vi "Apply Ethernet Configuration.vi"(7 "Restart (T)":bool=TRUE, 8 "error in (no error)":errorcluster, 10 "Ethernet Settings":T1={"IP Address"="192.168.1.100", "TCP (Command) Port"=12345, "TCP (Command) Read Interval (ms)"=10, "UDP (Reporting) Port"=54321, "UDP (Reporting) Write Interval (ms)"=5, "UDP Data Broadcast Enable"=FALSE}, 11 "Ethernet in":refnum<class "ENET_BS120x.lvclass">) -> (0 "error out":errorcluster, 3 "Ethernet out":refnum<class "ENET_BS120x.lvclass">)   [LabVIEW 2021, in "BS120x Driver.lvlib" / "ENET_BS120x.lvclass"]
doc: "Sends the configuration updates to the Battery Simulator 1200, and automatically triggers a restart.\nFor BS1201: the Restart input is no longer required. Restart is automatic on the BS1201 when configuration changes are made.\n(c) 2019 Bloomy Controls, Inc. All rights reserved."
uses:
  ENET_BS120x.lvclass
  TypeDefs/Ethernet Settings.ctl
  ENET_BS120x.lvclass/ENET_BS120x.ctl
  BS120x.lvclass
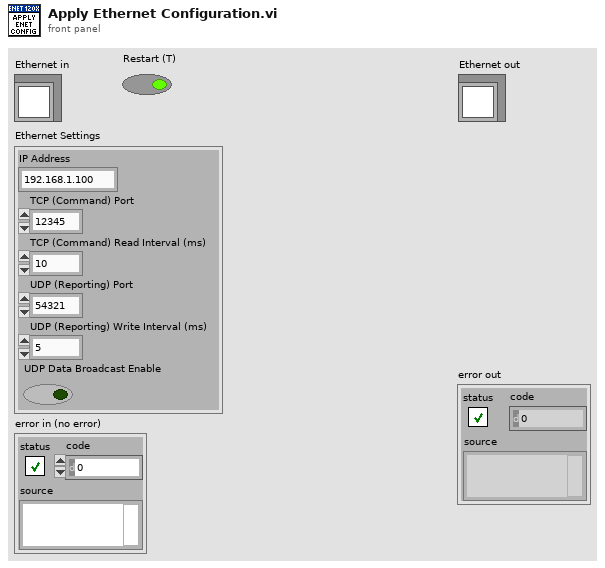
[diagram p1: front panel]
types:
  T1 = typedef "BS120x Driver.lvlib/BS120x.lvclass/Ethernet Settings.ctl" = cluster{"IP Address":string, "TCP (Command) Port":u16, "TCP (Command) Read Interval (ms)":u32, "UDP (Reporting) Port":u16, "UDP (Reporting) Write Interval (ms)":u32, "UDP Data Broadcast Enable":bool}
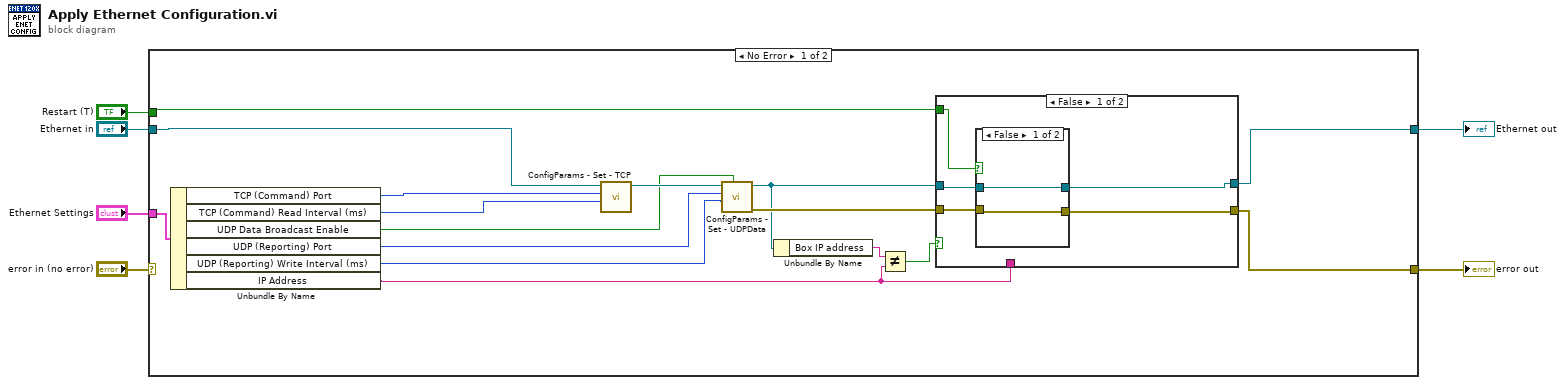
[diagram p0: block diagram]
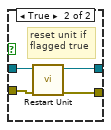
[diagram p2: hidden frame]
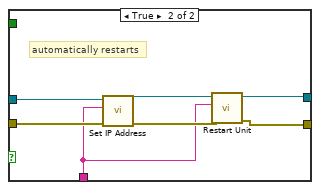
[diagram p3: hidden frame]
diagram:
  n1 = case shown="No Error" "error in (no error)" {
    selector: "error in (no error)" -> [_ w42]
    tunnel: [w13 w42] -> w5
    tunnel: [w12 w41] -> w3
    tunnel: "Ethernet in" -> [w21 w41]
    tunnel: "Ethernet Settings" -> [w22 _]
    tunnel: "Restart (T)" -> [w7 _]
    frame No Error {
      n2 = Unbundle By Name(w22) -> ("TCP (Command) Port"=w20:u16, "TCP (Command) Read Interval (ms)"=w19:u32, "UDP Data Broadcast Enable"=w16:bool, "UDP (Reporting) Port"=w17:u16, "UDP (Reporting) Write Interval (ms)"=w15:u32, "IP Address"=w9:string)
      n3 = call-dynamic "ConfigParams - Set - TCP.vi"("TCPLoopTime_mS"=w19, "TCPCommandPort"=w20, "Ethernet in"=w21) -> ("Ethernet out"=w18:refnum<class "ENET_BS120x.lvclass">)  [unwired: 7 in, 1 out]
      n4 = call-dynamic "ConfigParams - Set - UDPData.vi"("UDP Data Enable"=w16, "UDPDataPeriod_mS"=w15, "UDP Data Port"=w17, "Ethernet in"=w18) -> ("error out"=w14:errorcluster, "Ethernet out"=w11:refnum<class "ENET_BS120x.lvclass">)  [unwired: 6 in]
      n5 = Unbundle By Name(w11) -> ("Box IP address"=w10:string)
      n6 = Not Equal?(x=w10, y=w9) -> (x != y?=w8:bool)
      n7 = case shown="False" w8 {
        tunnel: w14 -> [w27 w40]
        tunnel: w11 -> [w26 w39]
        tunnel: w9 -> [_ w36]
        tunnel: [w24 w34] -> w13
        tunnel: [w25 w35] -> w12
        tunnel: w7 -> [w23 _]
        frame False {
          n8 = case shown="False" w23 {
            tunnel: w27 -> [w28 w31]
            tunnel: w26 -> [w29 w33]
            tunnel: [w29 w32] -> w25
            tunnel: [w28 w30] -> w24
            frame False {
            }
            frame True {
              # "reset unit if\nflagged true"
              n9 = call-dynamic "Restart Unit.vi"("error in (no error)"=w31, "ENET in"=w33) -> ("error out"=w30:errorcluster, "ENET out"=w32:refnum<class "ENET_BS120x.lvclass">)  [unwired: 8 in]
            }
          }
        }
        frame True {
          # "automatically restarts"
          n10 = call-dynamic "Set IP Address.vi"("error in (no error)"=w40, "IP Address"=w36, "ENET in"=w39) -> ("error out"=w38:errorcluster, "ENET out"=w37:refnum<class "ENET_BS120x.lvclass">)  [unwired: 7 in]
          n11 = call-dynamic "Restart Unit.vi"("error in (no error)"=w38, "New IP (empty = original)"=w36, "ENET in"=w37) -> ("error out"=w34:errorcluster, "ENET out"=w35:refnum<class "ENET_BS120x.lvclass">)  [unwired: 7 in]
        }
      }
    }
    frame Error {
    }
  }
  "error out" <- w5
  "Ethernet out" <- w3
